vi "STA - Wave V5 Host_Wait.vi"() -> ()   [LabVIEW 2015]
doc: "The continuous acquisition mode tells the FPGA to acquire points indefinitely until a stop command is issued or until an error is encountered (FIFO overflow, module underflow, and so on). \n\nIn this acquisition mode, explicitly call the appropriate rwfm_ConfigTiming VI and set the host application's data buffer to be many times larger than the read size. The examples use a 10X size by default. If the host application's data buffer fills, then the FPGA experiences a FIFO overflow causing the acquisition to stop."
uses:
  <vilib>/LabVIEW Targets/FPGA/cRIO/shared/nicrio_ModuleControls/nicrio_cRIO-9234_ConfigModeRing.ctl
  <vilib>/FPGAPlugInAG/cRIO-9112/niLvFpga_Open_cRIO-9112.vi
  <vilib>/rvi/interface/common/dynamic/niFpgaDynamicAddResources.vi
  <vilib>/Utility/error.llb/Error Cluster From Error Code.vi
  <vilib>/RVI Host/nirviSupport.llb/nirviErrorClusterFromErrorCode.vi
  <vilib>/rvi/errors/niLvFpgaAdjustHostInterfaceError.vi
  <vilib>/FPGAPlugInAG/Dynamic/niLvFpga_Close_Dynamic.vi
  <vilib>/rvi/interface/nirviOpenFPGA/nirviOpenFPGA.xnode
  FPGA Bitfiles/STA-WaveformV5_FPGATarget2_[FPGA]DeltaSigMa_sLRIAVfzKK0.lvbitx
  FPGA/[FPGA] DeltaSig Main V5.vi
  <vilib>/rvi/interface/nirviMethod/nirviMethod.xnode
  <vilib>/rvi/interface/nirviCloseFPGA/nirviCloseFPGA.xnode
  <vilib>/NI/cRIO Wfm/cRIO Wfm.lvlib
  <vilib>/rvi/interface/nirviMethod/StockFPGA_InlinedMethodWaitForSingleIRQ.vi
  <vilib>/FPGAPlugInAG/Dynamic/niLvFpga_WaitOnIrq_Dynamic.vi
  C:/Program Files (x86)/National Instruments/LabVIEW 2015/ProjectTemplates/Source/cRIOWfm/FPGA/[FPGA] SAR Acq Main.vi
  D/Documents/LabVIEW Data/STA - Waveform V0/FPGA Bitfiles/SARAcqMain_9074.lvbitx
panel:
  out "time stamp":timestamp
  out "Waveform Data":waveform(sgl)[](array[waveform])
  in  "base path":path=path "u:/"
  out "Time Measure":dbl
  out "data rate (S/s)":u32
  out "Channel Config":T2(array[cluster]) {"Input Configuration" items=["AC Coupled", "DC Coupled", "IEPE AC Coupled"]}
  in  "Samples per Read":i32=10000
  out "file path":path
  out "error out":errorcluster
  in  "stop":bool
  out "Waveform Graph":waveform(sgl)[](graph)
  out "Buffer Backlog":dbl caption="RT Buffer Backlog [%]" format="%#.2g"
  # "Sampling Info"
  # "Channel Info"
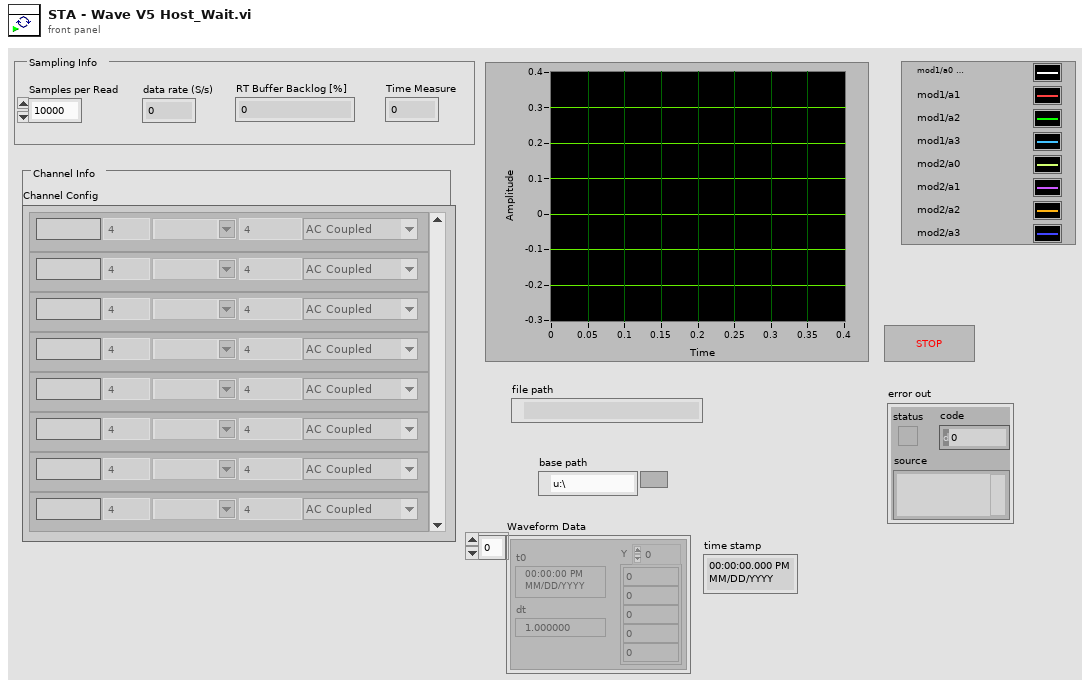
[diagram p1: front panel]
types:
  T1 = typedef "nicrio_cRIO-9234_ConfigModeRing.ctl" = u8
  T2 = cluster{"Channel Name":string, "Sensitivity mV_EU":dbl, "EU":string, "Input Configuration":T1, "dB Ref EU":dbl}[]
  T3 = enum16{"open", "open or create", "create or replace", "create", "open (read-only)"}
  T4 = typedef "Acquisition and Logging Configuration_Waveform.ctl" = cluster{"Samples per Read":i32, "Number of Reads to Save":i32, "Data File Name":string, "TDMS Properties":T5[], "Number of Channels":i32, "Trigger - RMS Value":dbl, "Trigger - Channel":i32, "Trigger - Time (Minute)":i32, "Channel Config":cluster{"Channel Name":string, "Sensitivity mV_EU":dbl, "EU":string, "Input Configuration":T1, "dB Ref EU":dbl}[], "data rate (S/s)":u32, "Time Measure":dbl}
  T5 = typedef "TDMS Properties.ctl" = cluster{"Name":string, "Value":string}
  T6 = typedef "cRIO Wfm.lvlib/SamplingInfo.ctl" = cluster{"Number of Channels":i32, "Actual Samp Rate":dbl, "Chan Name Array":string[], "EU Chan Array":string[], "dB Ref Chan Array":dbl[]}
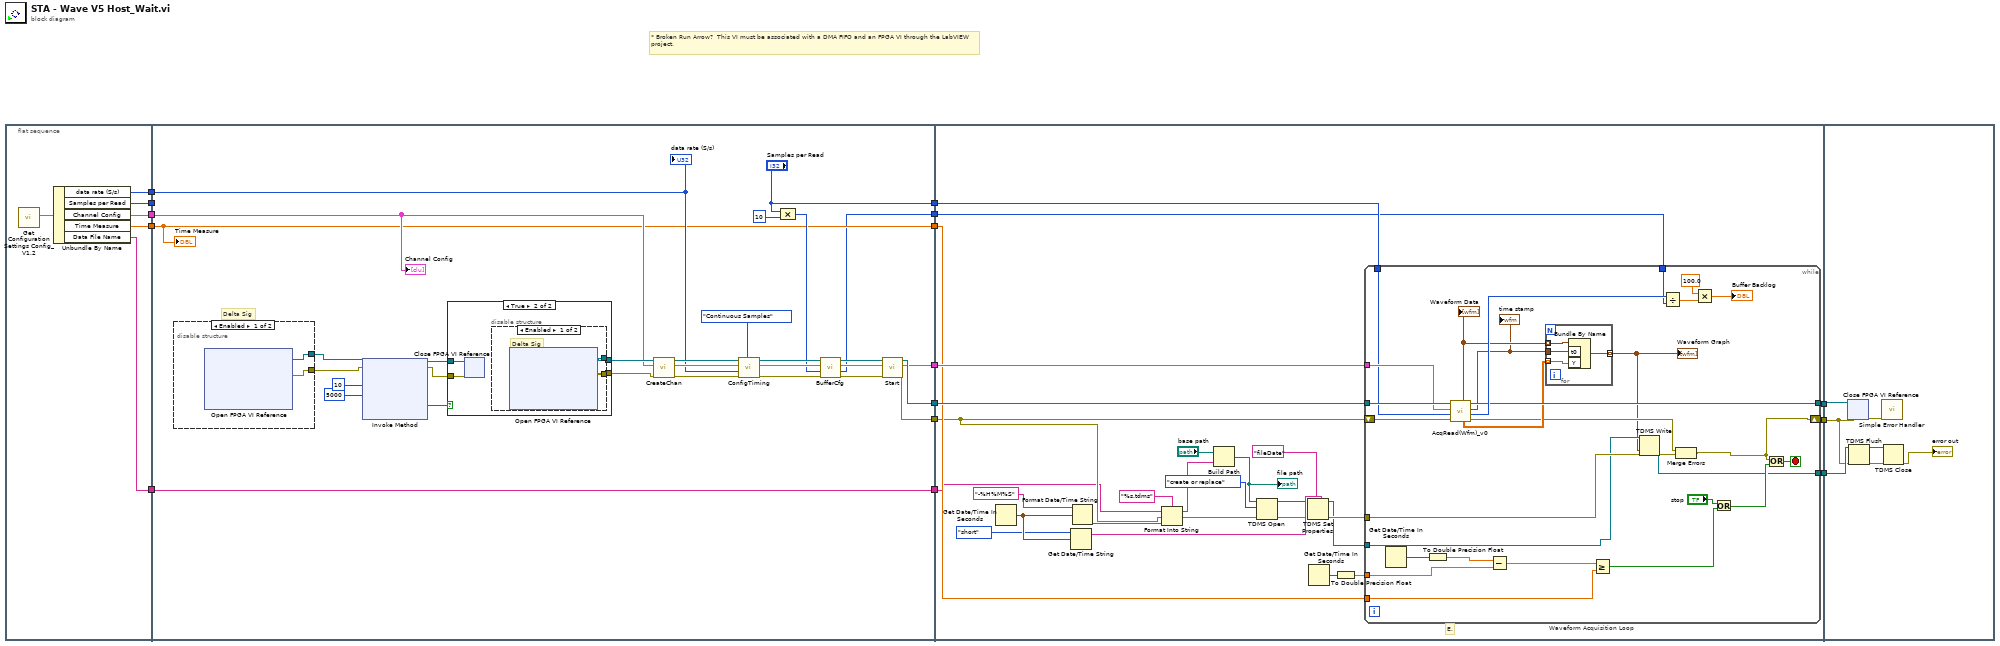
[diagram p0: block diagram]
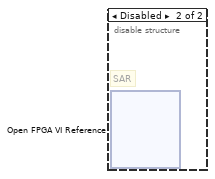
[diagram p2: hidden frame]
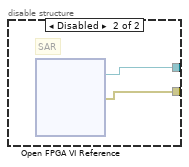
[diagram p4: hidden frame]
diagram:
  # "* Broken Run Arrow?  This VI must be associated with a DMA FIFO and an FPGA VI through the LabVIEW project."
  n1 = flat-sequence {
    tunnel: [w20] -> w15
    tunnel: [w19] -> w14
    tunnel: [w18] -> w13
    tunnel: [w17] -> w12
    tunnel: [w16] -> w2
    tunnel: w15 -> [w32]
    tunnel: w14 -> [_]
    tunnel: w13 -> [w31]
    tunnel: w12 -> [w24]
    tunnel: ["Samples per Read"] -> w11
    tunnel: [w24] -> w10
    tunnel: [w28] -> w9
    tunnel: [w27] -> w8
    tunnel: [w26] -> w7
    tunnel: [w23] -> w6
    tunnel: w2 -> [w22]
    tunnel: [w22] -> w1
    tunnel: w11 -> [w70]
    tunnel: w10 -> [w72]
    tunnel: w9 -> [w74]
    tunnel: w8 -> [w73]
    tunnel: w7 -> [w68]
    tunnel: w6 -> [w69]
    tunnel: [w77] -> w5
    tunnel: [w76] -> w4
    tunnel: [w75] -> w3
    tunnel: w1 -> [w66]
    tunnel: w5 -> [w129]
    tunnel: w4 -> [w127]
    tunnel: w3 -> [w128]
    frame #0 {
      n2 = call "Get Configuration Settings Config_V1.2.vi"() -> ("Configuration"=w21:T4)  [unwired: 10 in, 1 out]
      n3 = Unbundle By Name(w21) -> ("data rate (S/s)"=w20:u32, "Samples per Read"=w19:i32, "Channel Config"=w18:T2, "Time Measure"=w17:dbl, "Data File Name"=w16:string)
    }
    frame #1 {
      # "Delta Sig"
      n4 = disable-structure shown="Enabled" {
        disable-tunnel: [w53 _] -> w30
        disable-tunnel: [w52 _] -> w29
        frame Enabled {
          n5 = xnode "Open FPGA VI Reference"() -> ("FPGA VI Reference Out"=w53:refnum<k20>, "error out"=w52:errorcluster)  [unwired: 2 in]
        }
        frame Disabled {
          # "SAR"
          n6 = xnode "Open FPGA VI Reference"() -> ("FPGA VI Reference Out"=w55:refnum<k20>, "error out"=w54:errorcluster)  [unwired: 2 in]
        }
      }
      n7 = xnode "Invoke Method"("FPGA VI Reference In"=w30, "error in"=w29, "IRQ Number(s)"=10, "Timeout (ms)"=5000) -> ("FPGA VI Reference Out"=w48:refnum<k20>, "error out"=w49:errorcluster, "Timed Out"=w47:bool)  [unwired: 1 out]
      n8 = case shown="True" w47 {
        tunnel: w48 -> [w57 w61]
        tunnel: w49 -> [w56 w60]
        tunnel: [w57 w59] -> w51
        tunnel: [w56 w58] -> w50
        frame False {
        }
        frame True {
          n9 = xnode "Close FPGA VI Reference"("FPGA VI Reference In"=w61, "error in"=w60) -> ()  [unwired: 1 out]
          n10 = disable-structure shown="Enabled" {
            disable-tunnel: [w63 w65] -> w59
            disable-tunnel: [w62 w64] -> w58
            frame Enabled {
              # "Delta Sig"
              n11 = xnode "Open FPGA VI Reference"() -> ("FPGA VI Reference Out"=w63:refnum<k20>, "error out"=w62:errorcluster)  [unwired: 2 in]
            }
            frame Disabled {
              # "SAR"
              n12 = xnode "Open FPGA VI Reference"() -> ("FPGA VI Reference Out"=w65:refnum<k20>, "error out"=w64:errorcluster)  [unwired: 2 in]
            }
          }
        }
      }
      n13 = call <vilib>:"CreateChan.vi"("Dynamic FPGA Ref"=w51, "Channel Config"=w31, "error in"=w50) -> ("Dynamic FPGA Ref Out"=w38:refnum<k20>, "Sampling Info"=w39:T6, "error out"=w43:errorcluster)  [unwired: 5 in]
      n14 = call <vilib>:"ConfigTiming.vi"("Sample Mode"=enum16{"Finite Samples", "Continuous Samples"}."Continuous Samples", "error in"=w43, "Sample Rate"=w32, "Sampling Info In"=w39, "Dynamic FPGA Ref"=w38) -> ("error out"=w42:errorcluster, "Sampling Info Out"=w41:T6, "Dynamic FPGA Ref Out"=w40:refnum<k20>)  [unwired: 3 in, 1 out]
      n15 = Compound Arithmetic op=MULTIPLY("Samples per Read", 10 ("value")) -> (w36:i32)
      n16 = call <vilib>:"BufferCfg.vi"("error in"=w42, "Buffer Size [Samps per Chan]"=w36, "Sampling Info In"=w41, "Dynamic FPGA Ref"=w40) -> ("error out"=w35:errorcluster, "Buffer Size [Total Samples]"=w23:u32, "Sampling Info Out"=w37:T6, "Dynamic FPGA Ref Out"=w34:refnum<k20>)  [unwired: 4 out]
      n17 = call <vilib>:"Start.vi"("error in"=w35, "Sampling Info In"=w37, "Dynamic FPGA Ref"=w34) -> ("error out"=w26:errorcluster, "Sampling Info Out"=w27:T6, "Dynamic FPGA Ref Out"=w28:refnum<k20>)  [unwired: 6 out]
      "Channel Config" <- w31
      "data rate (S/s)" <- w32
      "Time Measure" <- w24
    }
    frame #2 {
      # "E."
      n18 = Get Date/Time In Seconds() -> (seconds since 1Jan1904=w90:timestamp)
      n19 = Get Date/Time String(date format (0)=enum16{"short", "long", "abbreviated"}."short", seconds (now)=w90) -> (date string=w93:string)  [unwired: 1 in, 1 out]
      n20 = Format Date/Time String(time format string (%c)="-%H%M%S", seconds (now)=w90) -> (date/time string=w81:string)  [unwired: 1 in]
      n21 = Format Into String(format string="%s.tdms", initial string=w66, error in=w68, w81) -> (resulting string=w78:string, error out=w87:errorcluster)
      n22 = Build Path(base path="base path", name or relative path=w78) -> (appended path=w84:path)
      "file path" <- w84
      n23 = TDMS Open(8:w87, 10:T3."create or replace" ("operation (0:open)"), 11:w84) -> (0:w82:errorcluster, 3:w83:refnum<k34>)  [unwired: 4 in]
      n24 = TDMS Set Properties(5:w93, 7:"fileDate" ("property names"), 8:w82, 11:w83) -> (0:w89:errorcluster, 3:w88:refnum<k34>)  [unwired: 2 in, 2 out]
      n25 = Get Date/Time In Seconds() -> (seconds since 1Jan1904=w92:timestamp)
      n26 = To Double Precision Float(number=w92) -> (double precision float=w91:dbl)
      n27 = while "Waveform Acquisition Loop" {
        tunnel: [w116] -> w77
        shift-right: [w111] -> w76
        shift-left: w68 -> [w122]
        tunnel: w88 -> [w97]
        tunnel: w89 -> [w98]
        tunnel: [w96] -> w75
        tunnel: w91 -> [w104]
        tunnel: w72 -> [w103]
        tunnel: w74 -> [w102]
        tunnel: w73 -> [w101]
        tunnel: w70 -> [w100]
        tunnel: w69 -> [w99]
        stop <- w117 stop-if-true
        n28 = Get Date/Time In Seconds() -> (seconds since 1Jan1904=w106:timestamp)
        n29 = To Double Precision Float(number=w106) -> (double precision float=w105:dbl)
        n30 = call <vilib>:"AcqRead(Wfm)_v0.vi"("error in"=w122, "Samps Read per Chan"=w100, "Sampling Info"=w101, "Dynamic FPGA Ref"=w102) -> ("error out"=w112:errorcluster, "Samples Remaining"=w121:u32, "time stamp"=w113:timestamp, "Dynamic FPGA Ref Out"=w116:refnum<k20>, "transposed array"=w114:sgl[][], "Array"=w115:waveform(sgl)[])  [unwired: 2 in]
        "Waveform Data" <- w115
        "time stamp" <- w113
        n31 = Subtract(x=w105, y=w104) -> (x-y=w107:dbl)
        n32 = for {
          tunnel: w115 -> [w126] mode=indexing
          tunnel: w113 -> [w125]
          tunnel: [w124] -> w95 mode=indexing
          tunnel: w114 -> [w123] mode=indexing
          n33 = Bundle By Name(cluster=w126, "t0"=w125, "Y"=w123) -> (w124:waveform(sgl))
        }
        "Waveform Graph" <- w95
        n34 = Greater Or Equal?(x=w107, y=w103) -> (x >= y?=w110:bool)
        n35 = TDMS Write(0:w97, 9:w95, 11:w98) -> (4:w96:refnum<k34>, 15:w94:errorcluster)  [unwired: 3 in, 2 out]
        n36 = Divide(x=w121, y=w99) -> (x/y=w120:dbl)
        n37 = Merge Errors(w112, w94) -> (w111:errorcluster)
        n38 = Multiply(x=100.0, y=w120) -> (x*y=→"Buffer Backlog":dbl)
        n39 = Or(x="stop", y=w110) -> (x .or. y?=w108:bool)
        n40 = Or(x=w111, y=w108) -> (x .or. y?=w117:bool)
      }
    }
    frame #3 {
      n41 = xnode "Close FPGA VI Reference"("FPGA VI Reference In"=w129, "error in"=w127) -> ("error out"=w130:errorcluster)
      n42 = TDMS Flush(4:w127, 7:w128) -> (0:w131:errorcluster, 3:w133:refnum<k34>)
      n43 = call <vilib>:"Simple Error Handler.vi"("error in (no error)"=w130) -> ()  [unwired: 1 in, 8 out]
      n44 = TDMS Close(8:w131, 11:w133) -> (0:→"error out":errorcluster)  [unwired: 1 out]
    }
  }
